vi "Write Monitor File.vi"(8 "error in (no error)":errorcluster, 9 "Open plot":bool, 10 "Monitor File":path, 11 "Monitor-Pulse in":refnum<class "Monitor-Pulse.lvclass">) -> (0 "error out":errorcluster, 3 "Monitor-Pulse out":refnum<class "Monitor-Pulse.lvclass">)   [LabVIEW 2015, in "Monitor-Pulse.lvclass"]
uses:
  Monitor-Pulse.lvclass
  Monitor-Pulse.lvclass/Monitor-Pulse.ctl
  Measure_core/Plots/Plot Messages/Add file Msg/Add file Msg.lvclass/Add file Msg.ctl
  <vilib>/ActorFramework/Message Enqueuer/Message Enqueuer.lvclass/Message Enqueuer.ctl
  Measure_core/Plots/Plot types.ctl
  <vilib>/ActorFramework/Message Enqueuer/Enqueue.vi
  <vilib>/ActorFramework/Message Priority Queue/Priority Enqueue.vi
  Measure_core/Plots/Plot Messages/Add file Msg/Add file Msg.lvclass
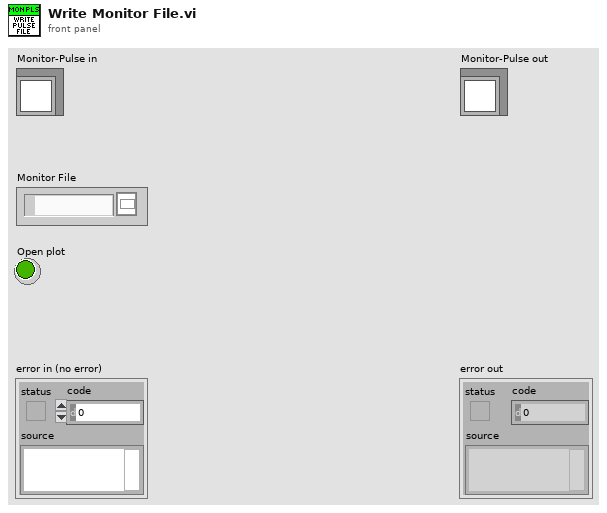
[diagram p1: front panel]
types:
  T1 = typedef "Plot types.ctl" = enum16{"Waveform Plot", "XY Plot", "Full XY"}
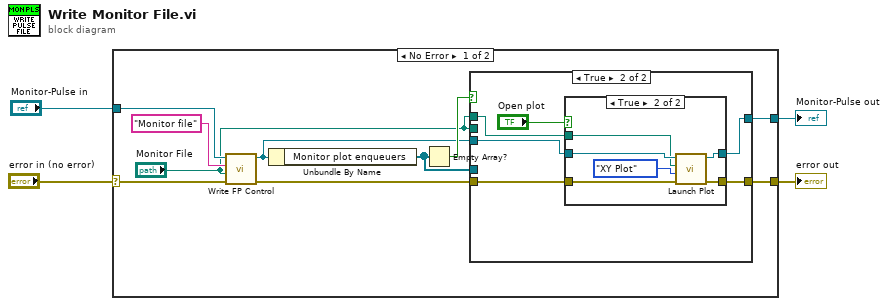
[diagram p0: block diagram]
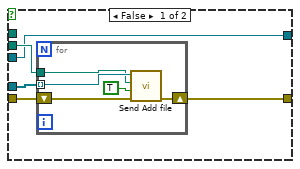
[diagram p2: hidden frame]
diagram:
  n1 = case shown="No Error" "error in (no error)" {
    selector: "error in (no error)" -> [w12 w40]
    tunnel: [w5 w40] -> w3
    tunnel: [w7 w39] -> w1
    tunnel: "Monitor-Pulse in" -> [w14 w39]
    frame No Error {
      n2 = call-dynamic "Write FP Control.vi"("error in (no error)"=w12, "Control Value"="Monitor File", "Control Name"="Monitor file", "Measure Object in"=w14) -> ("error out"=w6:errorcluster, "Measure Object out"=w8:refnum<class "Monitor-Pulse.lvclass">)  [unwired: 6 in]
      n3 = Unbundle By Name(w8) -> ("Monitor plot enqueuers"=w11:refnum<class "Message Enqueuer.lvclass">[])
      n4 = Empty Array?(array=w11) -> (empty?=w10:bool)
      n5 = case shown="True" w10 {
        tunnel: w6 -> [w17 w30]
        tunnel: [w16 w29] -> w5
        tunnel: w8 -> [w15 w28]
        tunnel: [w15 w27] -> w7
        tunnel: "Monitor File" -> [_ w26]
        tunnel: w11 -> [w19 _]
        tunnel: "Monitor File" -> [w18 _]
        frame False {
          n6 = for {
            tunnel: w19 -> [w24] mode=indexing
            tunnel: w18 -> [w23]
            shift-right: [w21] -> w16
            shift-left: w17 -> [w22]
            n7 = call "Send Add file.vi"("error in (no error)"=w22, "Insert in front"=TRUE, "File Path Control"=w23, "Message Enqueuer"=w24) -> ("error out"=w21:errorcluster)  [unwired: 6 in, 1 out]
          }
        }
        frame True {
          n8 = case shown="True" "Open plot" {
            tunnel: w30 -> [w32 w38]
            tunnel: [w32 w37] -> w29
            tunnel: w28 -> [w31 w36]
            tunnel: [w31 w35] -> w27
            tunnel: w26 -> [_ w34]
            frame False {
            }
            frame True {
              n9 = call-dynamic "Launch Plot.vi"("error in (no error)"=w38, "Plot type"=Plot_types."XY Plot", "File Path Control"=w34, "Monitor-Pulse in"=w36) -> ("error out"=w37:errorcluster, "Monitor-Pulse out"=w35:refnum<class "Monitor-Pulse.lvclass">)  [unwired: 5 in, 1 out]
            }
          }
        }
      }
    }
    frame Error {
    }
  }
  "error out" <- w3
  "Monitor-Pulse out" <- w1
